vi "Blinking_LED.vi"() -> ()   [LabVIEW 2020]
panel:
  in  "Button":bool
  out "Waveform Chart":i16(graph)
  out "Blinking LED":bool
  out "String":string
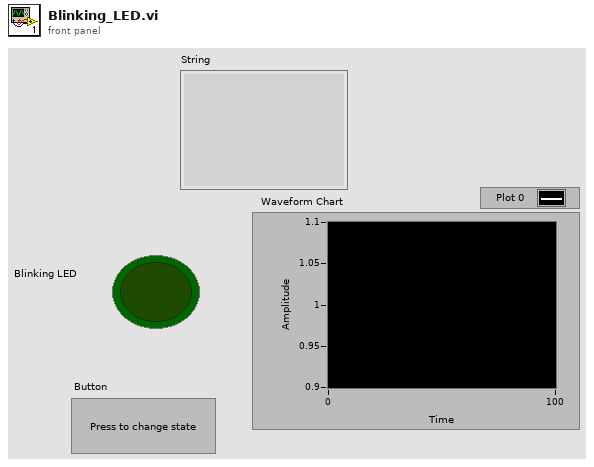
[diagram p1: front panel]
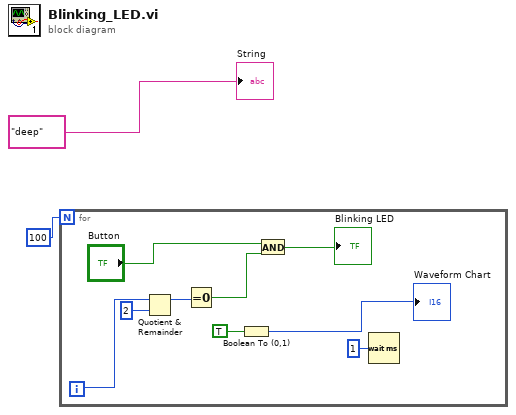
[diagram p0: block diagram]
diagram:
  n1 = for {
    N: 100 -> [_]
    i -> [w11]
    n2 = Quotient & Remainder(x=w11, y=2) -> (x-y*floor(x/y)=w9:i32)  [unwired: 1 out]
    n3 = Equal To 0?(x=w9) -> (x = 0?=w5:bool)
    n4 = Boolean To (0,1)(Boolean=TRUE) -> (0, 1=→"Waveform Chart":i16)
    n5 = And(x="Button", y=w5) -> (x .and. y?=→"Blinking LED":bool)
    n6 = Wait (ms)(milliseconds to wait=u32 1) -> ()  [unwired: 1 out]
  }
  "String" <- "deep" ("String")
